vi "ChannelSettingsQuery.vi"(8 "error in":errorcluster, 11 "T560Trigger in":refnum<class "T560Trigger.lvclass">) -> (0 "error out":errorcluster, 3 "T560Trigger out":refnum<class "T560Trigger.lvclass">)   [LabVIEW 2020, in "T560Trigger.lvclass"]
doc: "Prepare a command to query the channel settings"
uses:
  T560Trigger.lvclass
  C:/GEECS/Developers Version/source/Device Drivers/Highland T564 DDG/SupportLibraries/DeviceSpecific/HighlandT560Lib/T560ChannelClass/T560Channel.lvclass
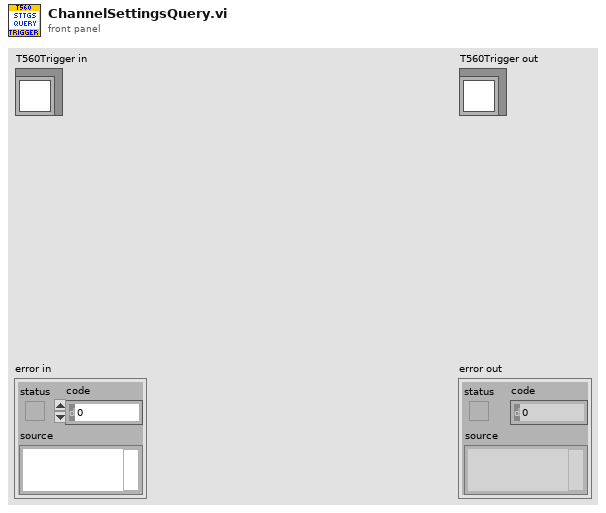
[diagram p1: front panel]
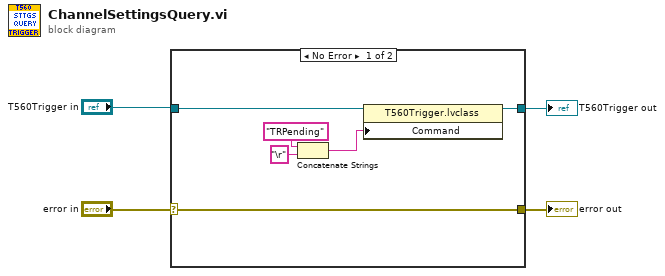
[diagram p0: block diagram]
diagram:
  n1 = case shown="No Error" "error in" {
    selector: "error in" -> [w10 w12]
    tunnel: [w10 w12] -> w2
    tunnel: [w6 w11] -> w1
    tunnel: "T560Trigger in" -> [w9 w11]
    frame No Error {
      n2 = Concatenate Strings("TRPending", "\r" ("string")) -> (w7:string)
      n3 = property class="T560Trigger.lvclass"(reference=w9, "Command"=w7) -> (reference out=w6:refnum<class "T560Trigger.lvclass">)  [unwired: 1 in, 1 out]
    }
    frame Error {
    }
  }
  "error out" <- w2
  "T560Trigger out" <- w1
